vi "Create Table Database.vi"(8 "error in (no error)":errorcluster, 11 "Contabilidad in":refnum<class "Contabilidad.lvclass">) -> (0 "error out":errorcluster, 3 "Contabilidad out":refnum<class "Contabilidad.lvclass">)   [LabVIEW 2020, in "Contabilidad.lvlib" / "Contabilidad.lvclass"]
uses:
  Contabilidad.lvclass
  <vilib>/drjdpowell/SQLite Library/SQL Connection/Open (path).vi
  <vilib>/drjdpowell/SQLite Library/SQL Connection/Open (string).vi
  <vilib>/AdvancedString/Path To Command Line String.vi
  <vilib>/drjdpowell/SQLite Library/SQL Connection/Execute SQL (No results).vi
  <vilib>/drjdpowell/SQLite Library/SQL Connection/Connection.lvclass
  <vilib>/drjdpowell/SQLite Library/SQLite.lvlib
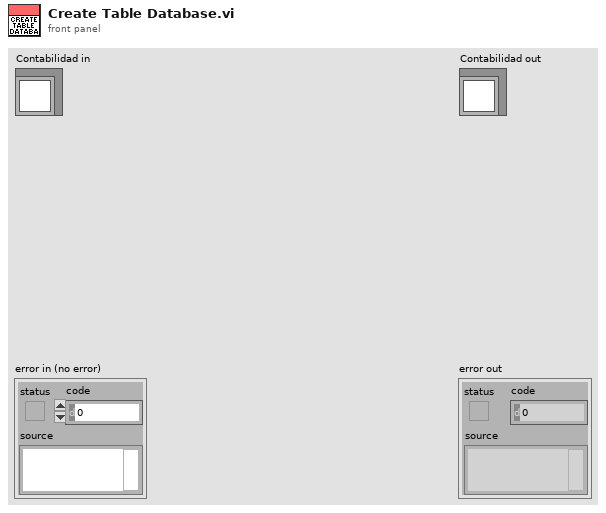
[diagram p1: front panel]
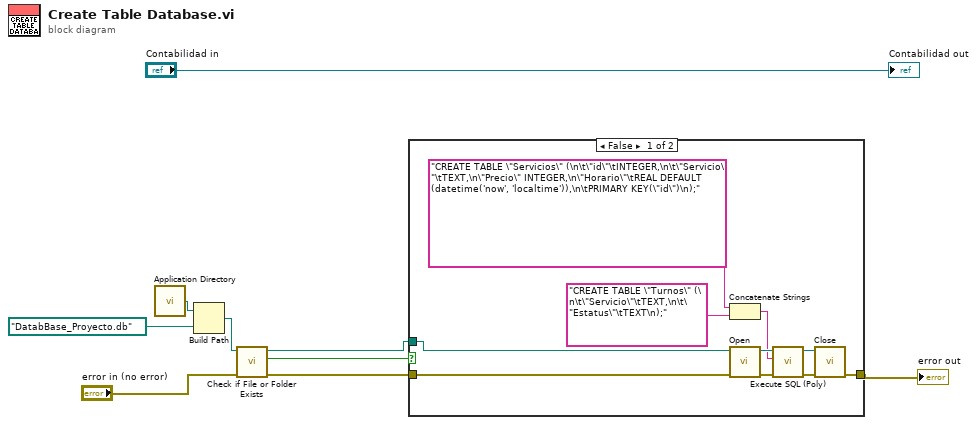
[diagram p0: block diagram]
diagram:
  n1 = call <vilib>:"Application Directory.vi"() -> ("Application Directory"=w5:path)
  n2 = Build Path(base path=w5, name or relative path=path "DatabBase_Proyecto.db") -> (appended path=w3:path)
  n3 = call <vilib>:"Check if File or Folder Exists.vi"("error in (no error)"="error in (no error)", "path"=w3) -> ("error out"=w6:errorcluster, "file or folder exists?"=w7:bool, "dup path"=w8:path)  [unwired: 7 in]
  n4 = case shown="False" w7 {
    tunnel: [w15 w20] -> w1
    tunnel: w8 -> [w13 _]
    tunnel: w6 -> [w14 w20]
    frame False {
      n5 = Concatenate Strings("CREATE TABLE \"Servicios\" (\n\t\"id\"\tINTEGER,\n\t\"Servicio\"\tTEXT,\n\"Precio\" INTEGER,\n\"Horario\"\tREAL DEFAULT (datetime('now', 'localtime')),\n\tPRIMARY KEY(\"id\")\n);", "CREATE TABLE \"Turnos\" (\n\t\"Servicio\"\tTEXT,\n\t\"Estatus\"\tTEXT\n);") -> (w10:string)
      n6 = call-poly <vilib>:"Open.vi"("error in (no error)"=w14, "db file"=w13) -> ("error out"=w19:errorcluster, "SQLite Connection"=w18:refnum<class "Connection.lvclass">)  [unwired: 8 in]
      n7 = call-poly <vilib>:"Execute SQL (Poly).vi"("error in (no error)"=w19, "SQL"=w10, "SQLite Connection in"=w18) -> ("error out"=w17:errorcluster, "SQLite Connection"=w16:refnum<class "Connection.lvclass">)  [unwired: 7 in]
      n8 = call-dynamic "Close.vi"("error in (no error)"=w17, "SQLite Connection in"=w16) -> ("error out"=w15:errorcluster)  [unwired: 9 in]
    }
    frame True {
    }
  }
  "error out" <- w1
  "Contabilidad out" <- "Contabilidad in"
